vi "Filter PDB XNodes.vi"(11 "References":refnum<vi>[](array[refnum])) -> (3 "PDB XNodes":refnum<vi>[](array[refnum]))   [LabVIEW 2020, in "Parallel Diagram Block.xnode"]
uses:
  Parallel Diagram Block.xnode
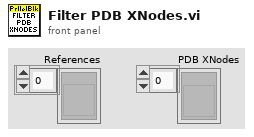
[diagram p1: front panel]
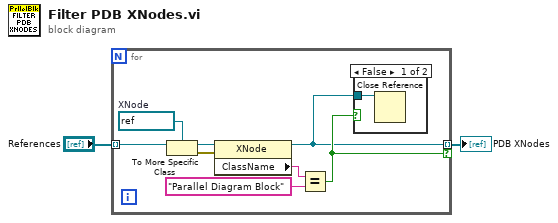
[diagram p0: block diagram]
diagram:
  n1 = for {
    tunnel: "References" -> [w10] mode=indexing
    tunnel: [w3] -> w1 mode=indexing if=w4
    w9 = refnum<vi> refnum  # XNode
    n2 = To More Specific Class(target class=w9, reference=w10) -> (specific class reference=w8:refnum<vi>, error out=w7:errorcluster)  [unwired: 1 in]
    n3 = property class="XNode"(reference=w8, error in=w7) -> (reference out=w3:refnum<vi>, "ClassName"=w6:string)  [unwired: 1 out]
    n4 = Equal?(x=w6, y="Parallel Diagram Block") -> (x = y?=w4:bool)
    n5 = case shown="False" w4 {
      tunnel: w3 -> [w11 _]
      frame False {
        n6 = Close Reference(reference=w11) -> ()  [unwired: 1 in, 1 out]
      }
      frame True {
      }
    }
  }
  "PDB XNodes" <- w1
